vi "serial communication (licor).vi"(4 "time (global)":dbl, 5 "Fehler":errorcluster caption="error in", 6 "command":string, 7 "read buffer in":string, 8 "VISA resource out":refnum<visa-resource-name>) -> (0 "Fehler (Ausgang)":errorcluster caption="error out", 1 "Licor-output":string[](array[string]), 2 "read buffer out":string, 3 "VISA resource out 2":refnum<visa-resource-name>)   [LabVIEW 2010]
uses:
  Licor-Steuerung/HAGAR V/Licor-Control/control/Emulate Licor output GV.vi
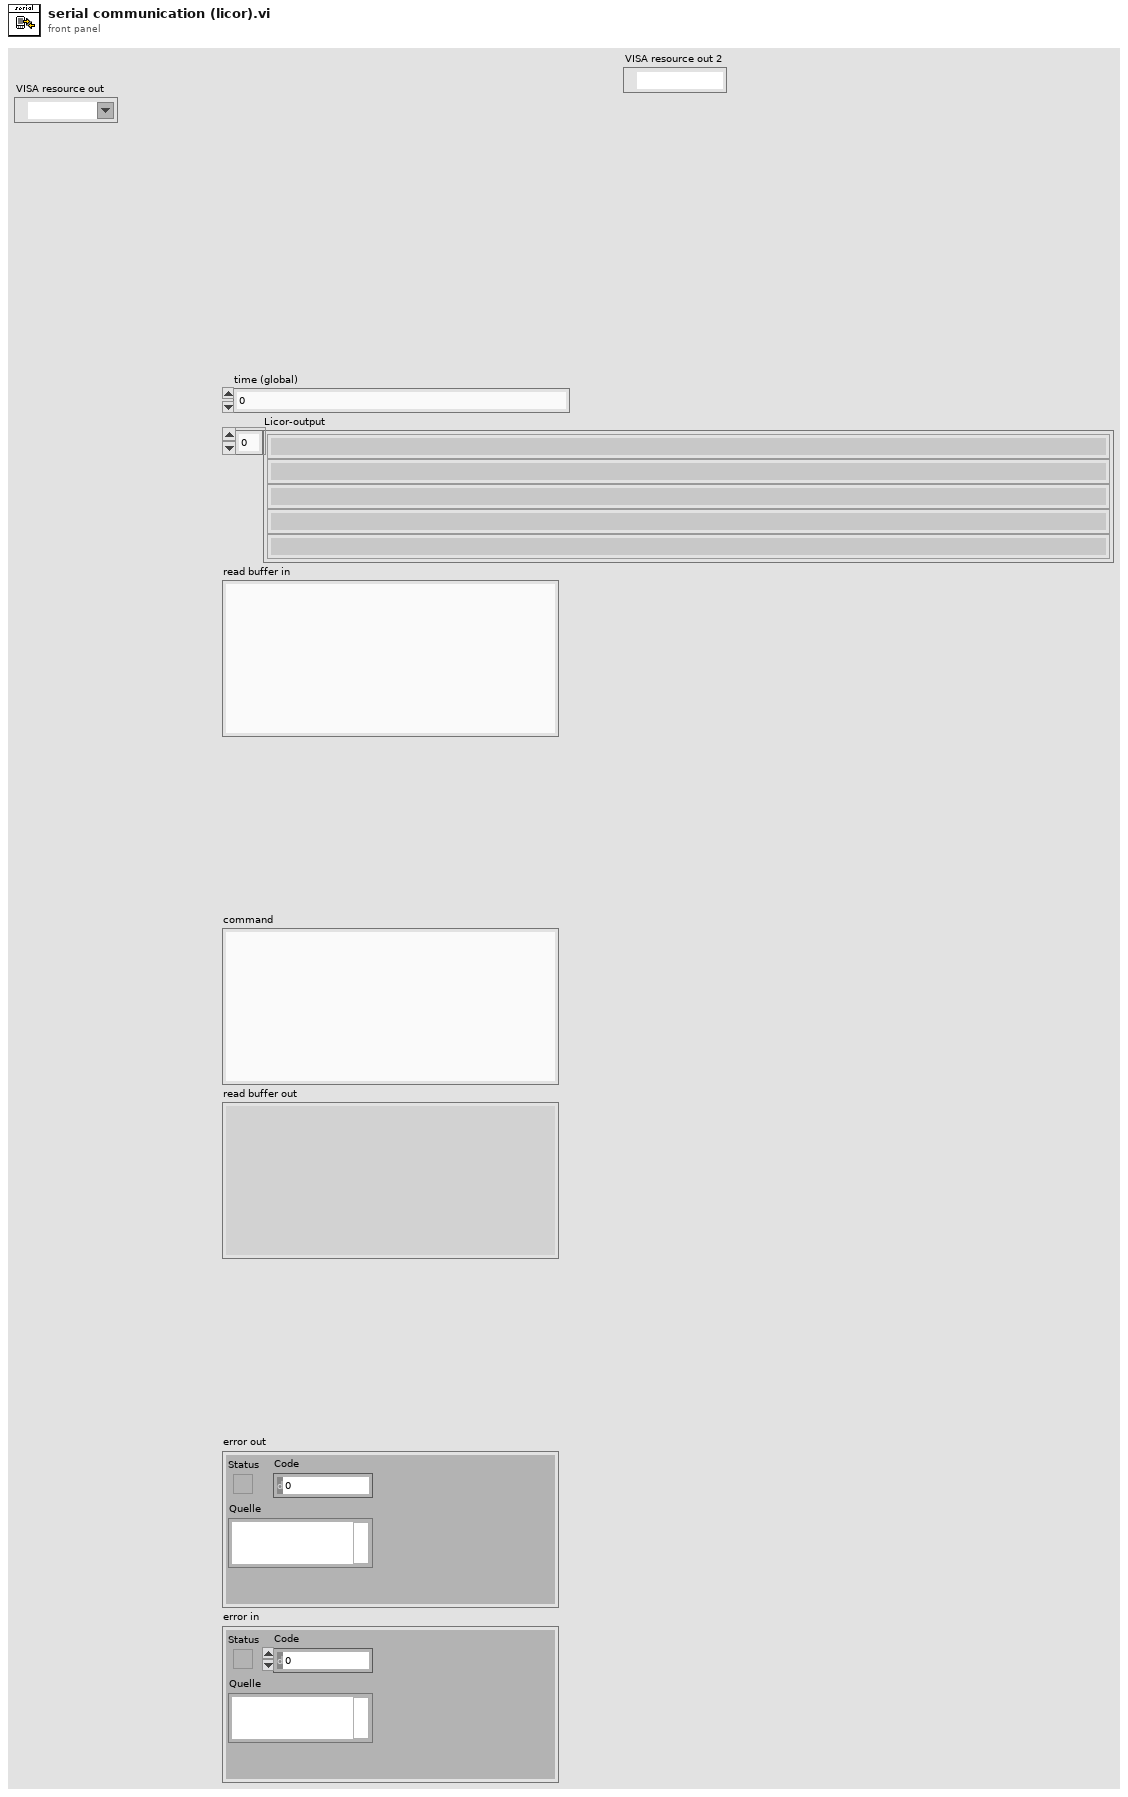
[diagram p1: front panel]
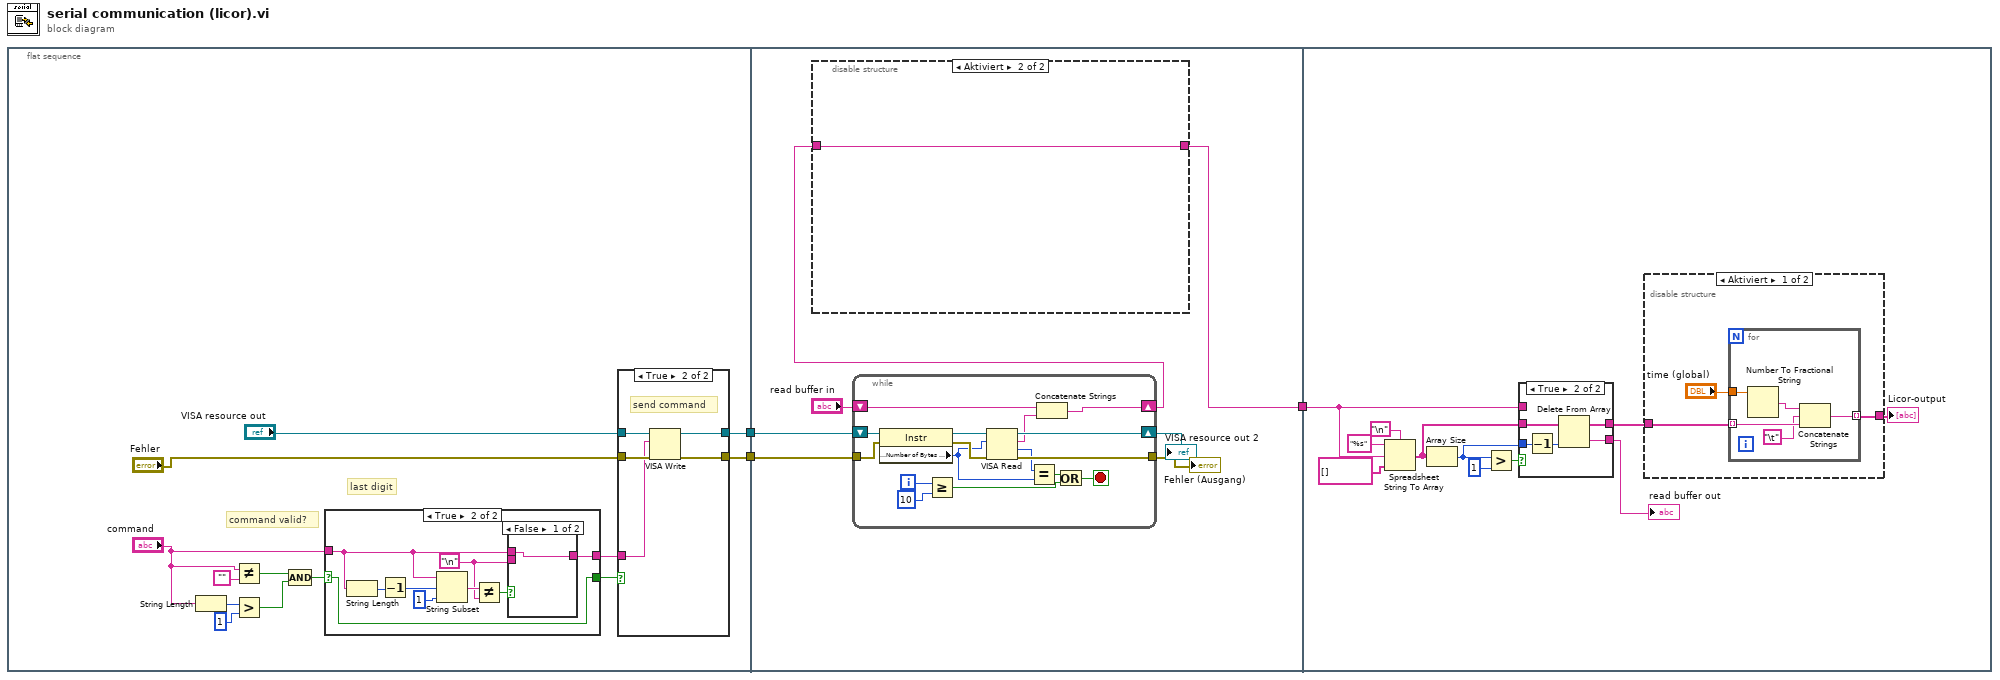
[diagram p0: block diagram]
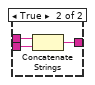
[diagram p4: hidden frame]
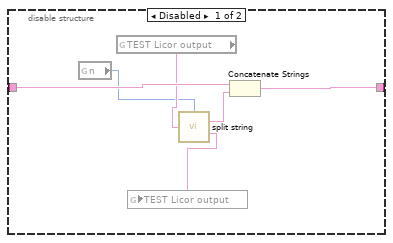
[diagram p5: hidden frame]
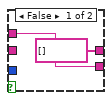
[diagram p7: hidden frame]
diagram:
  n1 = flat-sequence {
    tunnel: [w6] -> w2
    tunnel: [w5] -> w1
    tunnel: [w40] -> w3
    tunnel: w2 -> [w43]
    tunnel: w1 -> [w42]
    tunnel: w3 -> [w70]
    frame #0 {
      # "last digit"
      # "command valid?"
      n2 = String Length(string="command") -> (length=w9:i32)
      n3 = Not Equal?(x="command", y="") -> (x != y?=w8:bool)
      n4 = Greater?(x=w9, y=1) -> (0:w11:bool)
      n5 = Compound Arithmetic op=AND(w8, w11) -> (w12:bool)
      n6 = case shown="True" w12 {
        selector: w12 -> [w24 w27]
        tunnel: "command" -> [w25 w29]
        tunnel: [w25 w28] -> w16
        tunnel: [w24 w27] -> w14
        frame False {
        }
        frame True {
          w26 = "\n"
          n7 = String Length(string=w29) -> (length=w34:i32)
          n8 = Decrement(x=w34) -> (x-1=w33:i32)
          n9 = String Subset(string=w29, offset (0)=w33, length (rest)=1 ("Länge (Rest)")) -> (substring=w30:string)
          n10 = Not Equal?(x=w30, y=w26) -> (x != y?=w31:bool)
          n11 = case shown="False" w31 {
            tunnel: w29 -> [w35 w38]
            tunnel: w26 -> [_ w37]
            tunnel: [w35 w36] -> w28
            frame False {
            }
            frame True {
              n12 = Concatenate Strings(w38, w37) -> (w36:string)
            }
          }
        }
      }
      n13 = case shown="True" w14 {
        tunnel: "VISA resource out" -> [w18 w23]
        tunnel: "Fehler" -> [w17 w22]
        tunnel: w16 -> [_ w21]
        tunnel: [w18 w20] -> w6
        tunnel: [w17 w19] -> w5
        frame False {
        }
        frame True {
          # "send command"
          n14 = VISA Write(VISA resource name=w23, write buffer=w21, error in (no error)=w22) -> (VISA resource name out=w20:refnum<visa-resource-name>, error out=w19:errorcluster)  [unwired: 1 out]
        }
      }
    }
    frame #1 {
      n15 = while {
        shift-right: [w68] -> w39
        shift-left: w43 -> [w58]
        tunnel: [w67] -> w44
        shift-right: [w66] -> w41
        shift-left: "read buffer in" -> [w65]
        tunnel: w42 -> [w55]
        i -> [w63]
        stop <- w59 stop-if-true
        n16 = property class="Instr"(reference=w58, error in=w55) -> (reference out=w57:refnum<visa-resource-name>, error out=w56:errorcluster, "Serial Settings:Number of Bytes at Serial Port"=w54:u32)
        n17 = Greater Or Equal?(x=w63, y=10) -> (x >= y?=w60:bool)
        n18 = VISA Read(VISA resource name=w57, byte count=w54, error in (no error)=w56) -> (VISA resource name out=w68:refnum<visa-resource-name>, read buffer=w53:string, return count=w64:u32, error out=w67:errorcluster)
        n19 = Equal?(x=w64, y=w54) -> (x = y?=w61:bool)
        n20 = Concatenate Strings(w65, w53) -> (w66:string)
        n21 = Or(x=w61, y=w60) -> (x .or. y?=w59:bool)
      }
      "Fehler (Ausgang)" <- w44
      "VISA resource out 2" <- w39
      n22 = disable-structure shown="Aktiviert" {
        disable-tunnel: w41 -> [w51 w52]
        disable-tunnel: [w50 w52] -> w40
        frame Disabled {
          n23 = global read "Emulate Licor output GV.vi" "n"() -> (w46:i32)
          n24 = global read "Emulate Licor output GV.vi" "TEST Licor output"() -> (w48:string)
          n25 = call "split string.vi"("Index i"=w46, "String"=w48) -> ("out 1 (0 bis i-1)"=w49:string, "out 2 (i bis n)"=w47:string)  [unwired: 12 in]
          n26 = global write "Emulate Licor output GV.vi" "TEST Licor output"(w47) -> ()
          n27 = Concatenate Strings(w51, w49) -> (w50:string)
        }
        frame Enabled {
        }
      }
    }
    frame #2 {
      n28 = Spreadsheet String To Array(delimiter (Tab)="\n", format string="%s", spreadsheet string=w70, array type (2D Dbl)=string[] []) -> (array=w77:string[])
      n29 = Array Size(array=w77) -> (size(s)=w78:i32)
      n30 = Greater?(x=w78, y=1) -> (0:w79:bool)
      n31 = case shown="True" w79 {
        tunnel: w78 -> [_ w94]
        tunnel: w77 -> [_ w93]
        tunnel: [w90 w92] -> w69
        tunnel: w70 -> [w90 _]
        tunnel: [string[] [] w91] -> w71
        frame False {
        }
        frame True {
          n32 = Decrement(x=w94) -> (x-1=w95:i32)
          n33 = Delete From Array(array=w93, index=w95) -> (deleted portion=w92:string, array with subset deleted=w91:string[])  [unwired: 1 in]
        }
      }
      "read buffer out" <- w69
      n34 = disable-structure shown="Aktiviert" {
        disable-tunnel: [w82 w88] -> w72
        disable-tunnel: w71 -> [w81 w88]
        frame Enabled {
          n35 = for {
            tunnel: w81 -> [w86] mode=indexing
            tunnel: "time (global)" -> [w83]
            tunnel: [w84] -> w82 mode=indexing
            n36 = Number To Fractional String(number=w83) -> (F-format string=w87:string)  [unwired: 3 in]
            n37 = Concatenate Strings(w87, "\t", w86) -> (w84:string)
          }
        }
        frame Disabled {
        }
      }
      "Licor-output" <- w72
    }
  }
